vi "Read Micron Optics Driver.vi"(8 "error in (no error)":errorcluster, 11 "Micron Optics Recorder in":refnum<class "Micron Optics Recorder.lvclass">) -> (0 "error out":errorcluster, 2 "Micron Optics Driver.lvclass":refnum<class "Micron Optics Driver.lvclass">, 3 "Micron Optics Recorder out":refnum<class "Micron Optics Recorder.lvclass">)   [LabVIEW 2016, in "Micron Optics Recorder.lvclass"]
uses:
  Micron Optics Recorder.lvclass
  C:/github/Measure_core/Instrument Actor/Instrument Actor.lvclass
  NHMFL_Core/Libraries/Instruments/Micron Optics/Micron Optics Driver/Micron Optics Driver.lvclass
  Measure_core/Instrument Actor/Instrument Actor.lvclass/Instrument Actor.ctl
  Measure_core/Instrument Actor/Read Instrument driver.vi
  NHMFL_Core/Libraries/Instruments/Instrument Driver/Instrument Driver.lvclass
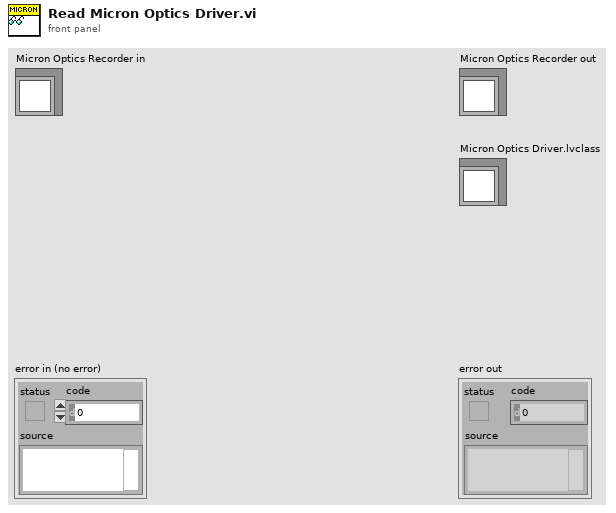
[diagram p1: front panel]
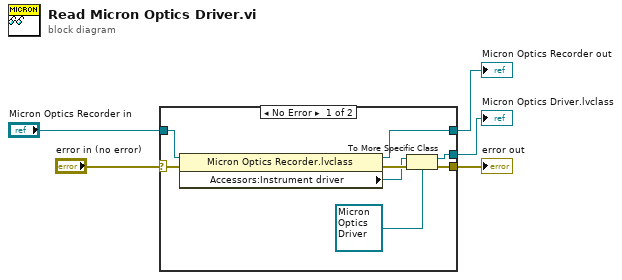
[diagram p0: block diagram]
diagram:
  n1 = case shown="No Error" "error in (no error)" {
    selector: "error in (no error)" -> [w13 w14]
    tunnel: [w9 w14] -> w4
    tunnel: [w10 w15] -> w2
    tunnel: "Micron Optics Recorder in" -> [w11 w15]
    tunnel: [w8 _] -> w1
    frame No Error {
      n2 = property class="Micron Optics Recorder.lvclass"(reference=w11, error in=w13) -> (reference out=w10:refnum<class "Micron Optics Recorder.lvclass">, error out=w12:errorcluster, "Accessors:Instrument driver"=w7:refnum<class "Instrument Driver.lvclass">)
      n3 = To More Specific Class(target class=refnum<class "Micron Optics Driver.lvclass"> refnum ("Micron Optics Driver.lvclass"), reference=w7, error in=w12) -> (specific class reference=w8:refnum<class "Micron Optics Driver.lvclass">, error out=w9:errorcluster)
    }
    frame Error {
    }
  }
  "error out" <- w4
  "Micron Optics Recorder out" <- w2
  "Micron Optics Driver.lvclass" <- w1
